vi "GetControls.vi"(6 "error in":errorcluster, 9 "Pane in":refnum<class "Pane.lvclass">) -> (0 "error out":errorcluster, 3 "Pane out":refnum<class "Pane.lvclass">, 4 "Controls":i32[](array[numeric]))   [LabVIEW 2014, in "Pane.lvclass"]
uses:
  Pane.lvclass
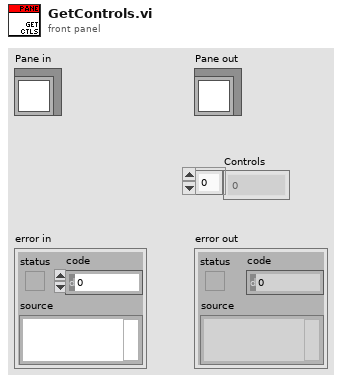
[diagram p1: front panel]
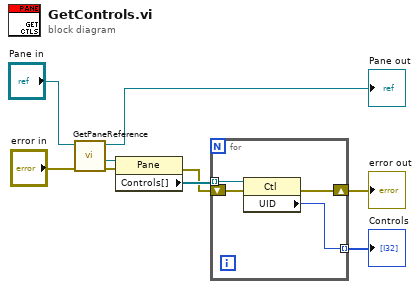
[diagram p0: block diagram]
diagram:
  n1 = call "GetPaneReference.vi"("error in"="error in", "Pane in"="Pane in") -> ("error out"=w3:errorcluster, "pane reference"=w4:refnum<vi>, "Pane out"=→"Pane out":refnum<class "Pane.lvclass">)  [unwired: 7 in]
  n2 = property class="Pane"(reference=w4, error in=w3) -> (error out=w1:errorcluster, "Controls[]"=w2:refnum<vi>[])  [unwired: 1 out]
  n3 = for {
    tunnel: w2 -> [w13] mode=indexing
    shift-right: [w11] -> w5
    shift-left: w1 -> [w12]
    tunnel: [w10] -> w6 mode=indexing
    n4 = property class="Ctl"(reference=w13, error in=w12) -> (error out=w11:errorcluster, "UID"=w10:i32)  [unwired: 1 out]
  }
  "error out" <- w5
  "Controls" <- w6
